vi "Release.vi"(8 "error in (no error)":errorcluster, 11 "Subscribe JSON in":refnum<class "Subscribe JSON.lvclass">) -> (0 "error out":errorcluster)   [LabVIEW 2020, in "wamplv.lvlib" / "Subscribe JSON.lvclass"]
uses:
  Subscribe JSON.lvclass
  Subscribe JSON.lvclass/Subscribe JSON.ctl
  fe5ca7f2-104d-4321-84dd-1908c4e8515b.vi
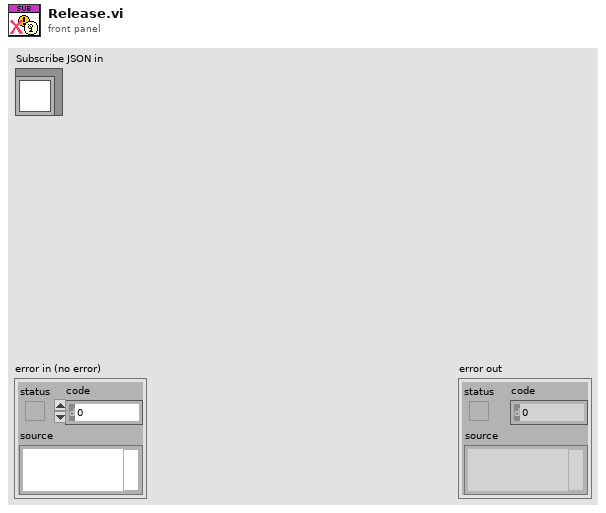
[diagram p1: front panel]
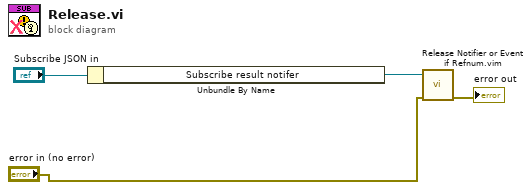
[diagram p0: block diagram]
diagram:
  n1 = Unbundle By Name("Subscribe JSON in") -> ("Subscribe result notifer"=w3:refnum<notifier>)
  n2 = call "Release Notifier or Event if Refnum.vim"("error in (no error)"="error in (no error)", "Notifier or Event in"=w3) -> ("error out"=→"error out":errorcluster)  [unwired: 9 in]
